vi "Main.vi"() -> ()   [LabVIEW 2020, in "SQSnobFit Control Panel.lvlib"]
uses:
  SQSnobFit Control Panel.lvlib
  process loops/Instrument Manager/Instrument State.ctl
  <vilib>/addons/zeromq/zmq_context.lvclass
  <vilib>/addons/zeromq/zmq_socket.lvclass
  process loops/UI Manager/support/Data Display Loop Data.ctl
  process loops/Logging/Logging Configuration.ctl
  process loops/UI Manager/support/UI Data.ctl
  process loops/UI Manager/support/UI Display State.ctl
  Typedefs/System Control Data.ctl
  <vilib>/Utility/error.llb/Error Cluster From Error Code.vi
  <vilib>/ErrorRing/Error Ring.xnode
  support/Message Queue/Message Queue.lvlib
  support/User Event - Stop/User Event - Stop.lvlib
  process loops/Instrument Manager/Instrument Manager.lvlib
  process loops/Acquisition/Acquisition.lvlib
  process loops/Remote Connection Manager/Remote Connection Manager.lvlib
  process loops/Logging/Logging.lvlib
panel:
  out "Next suggested parameters (percent)":cluster{"Name":string, "Value":dbl}[](array[cluster])
  in  "Overall Flow Rate (mL/min)":dbl format="%.3f"
  out "Next suggested parameters (values)":cluster{"Name":string, "Value":dbl}[](array[cluster])
  out "Response":string
  out "Optimizer Path":path
  in  "Time Interval (sec)":i32=1200
  out "Data Graph":cluster{timestamp[], dbl[]}[](graph)
  in  "Config Log Btn":bool
  in  "Sampling rate\n(sec/sample)":dbl=1.0 min=0.1 step=0.1
  in  "Log Data":bool
  in  "Submit Btn":bool
  in  "Yield":dbl format="%.3f"
  # "SQSnobFit"
  # "Optimizer Control"
  # "Config"
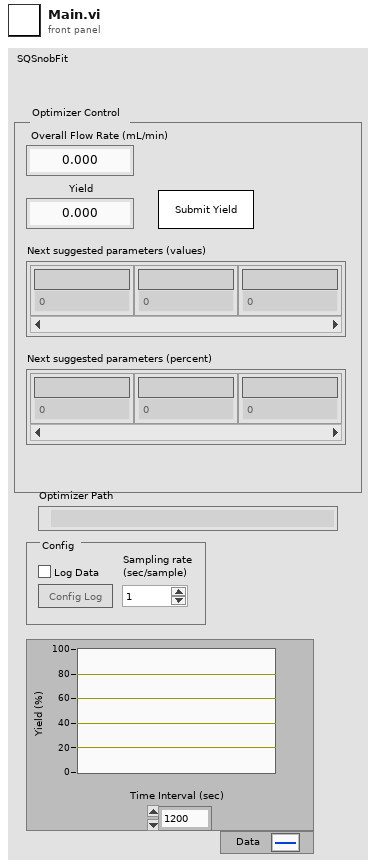
[diagram p1: front panel]
types:
  T1 = typedef "SQSnobFit Control Panel.lvlib/Data Display Loop Data.ctl" = cluster{"Data Timestamps":timestamp[], "Data Values":dbl[], "Previous Run State":bool}
  T2 = typedef "SQSnobFit Control Panel.lvlib/Instrument Manager.lvlib/Instrument State.ctl" = cluster{"Context":refnum<class "zmq_context.lvclass">, "Socket":refnum<class "zmq_socket.lvclass">, "Running Since":timestamp, "New Parameters (values)":cluster{"Time Stamp":timestamp, "Name":string[], "Value":dbl[]}, "Optimizer Path":path, "Running":bool, "Response Counter":u8, "Response Timeout (ms)":u32, "Response Retries":u32, "Endpoint":string, "Starting up?":bool, "New Parameters (percents)":cluster{"Time Stamp":timestamp, "Name":string[], "Value":dbl[]}, "Flow Rate Constant":dbl, "Yield":dbl, "Current Best (values)":cluster{"Parameter Names":string[], "Parameter Values":dbl[], "Function Value":dbl}}
  T3 = typedef "SQSnobFit Control Panel.lvlib/Message Queue.lvlib/All Message Queues.ctl" = cluster{"System Control":refnum<queue>, "Instrument":refnum<queue>, "Remote":refnum<queue>, "UI":refnum<queue>, "Acquisition":refnum<queue>, "Logging":refnum<queue>}
  T4 = typedef "SQSnobFit Control Panel.lvlib/UI Display State.ctl" = enum16{"Shown", "Hidden"}
  T5 = enum8{"Enabled", "Disabled", "Disabled and Grayed Out"}
  T6 = typedef "SQSnobFit Control Panel.lvlib/UI Data.ctl" = cluster{"Setpoint Ctl":refnum<vi>, "Submit Btn":refnum<vi>, "Log Data":refnum<vi>, "Config Log Btn":refnum<vi>, "Data Graph":refnum<vi>, "Flow Rate Ctl":refnum<vi>}
  T7 = typedef "SQSnobFit Control Panel.lvlib/Logging.lvlib/Logging Configuration.ctl" = cluster{"Log Directory Path":path, "Log File Path":path, "Log File Prefix":string, "Log File Extension":string, "File Delimiter":string, "Header Info":string[][], "Channels":string[], "Log Instrument Runs":bool}
  T8 = typedef "SQSnobFit Control Panel.lvlib/System Control Data.ctl" = cluster{"Example Value <Replace Me>":dbl, "Log Runs":bool, "Clone":bool}
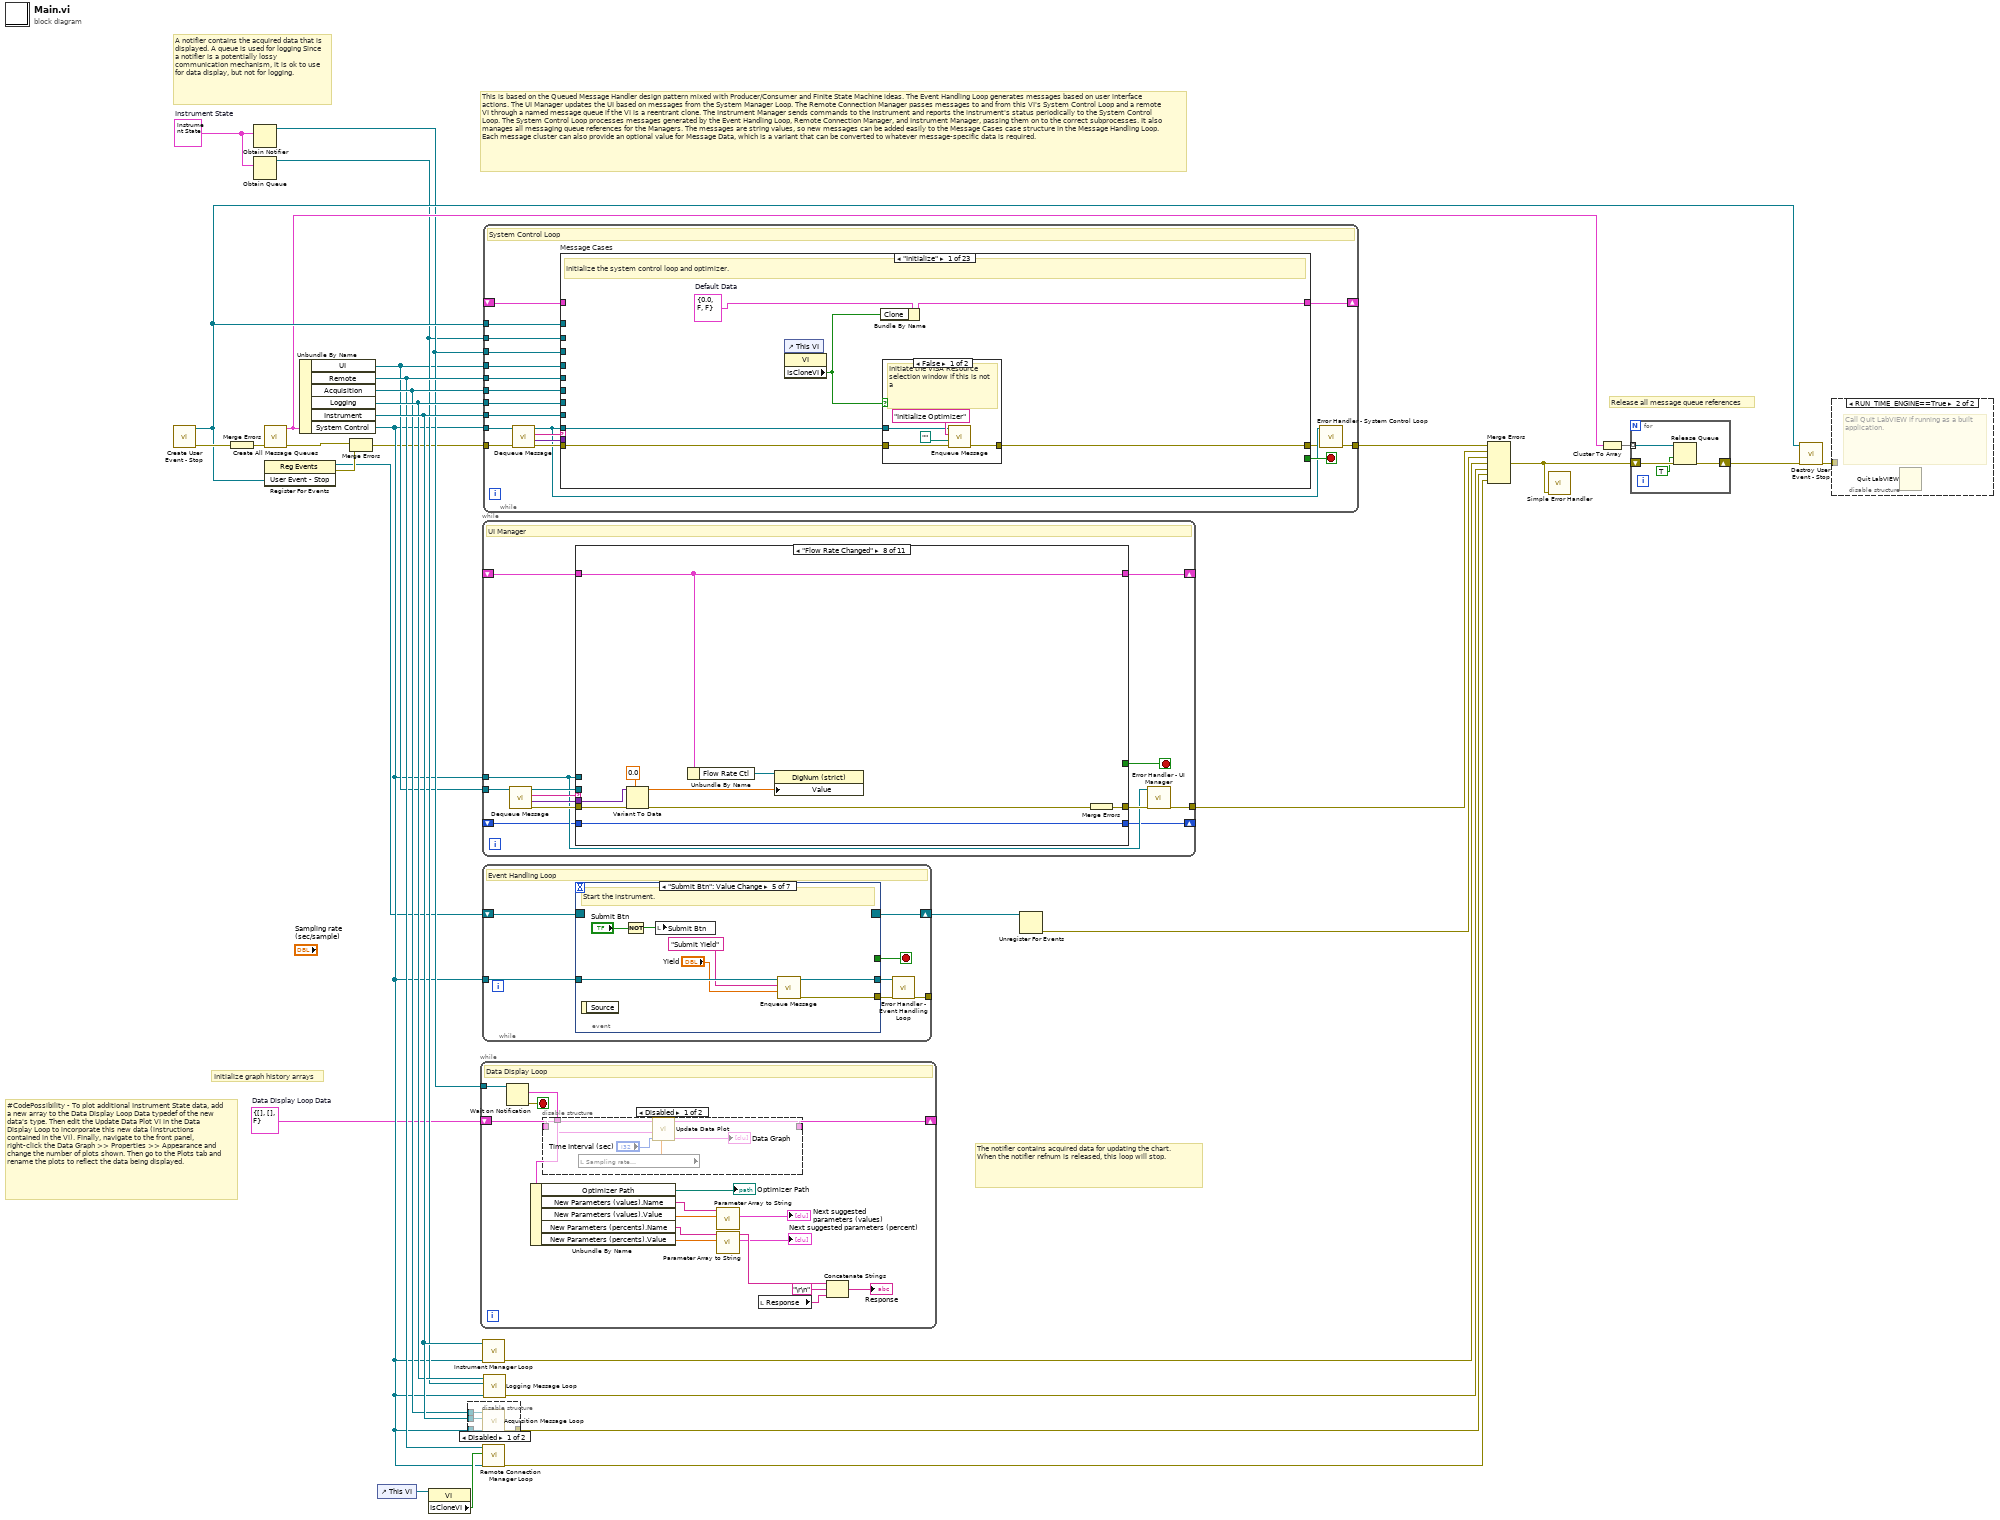
[diagram p0: block diagram]
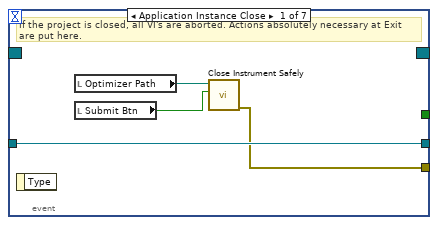
[diagram p4: hidden frame]
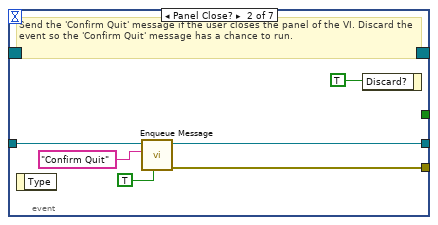
[diagram p5: hidden frame]
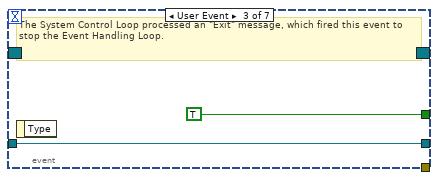
[diagram p6: hidden frame]
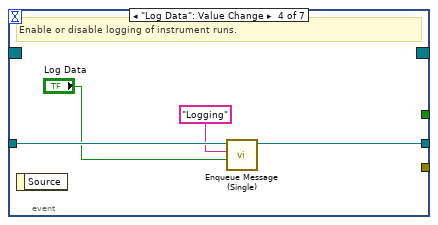
[diagram p7: hidden frame]
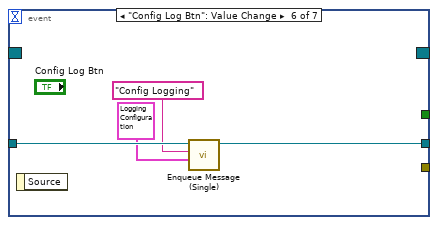
[diagram p8: hidden frame]
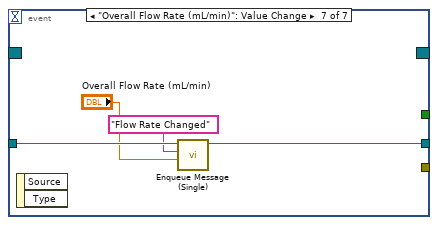
[diagram p9: hidden frame]
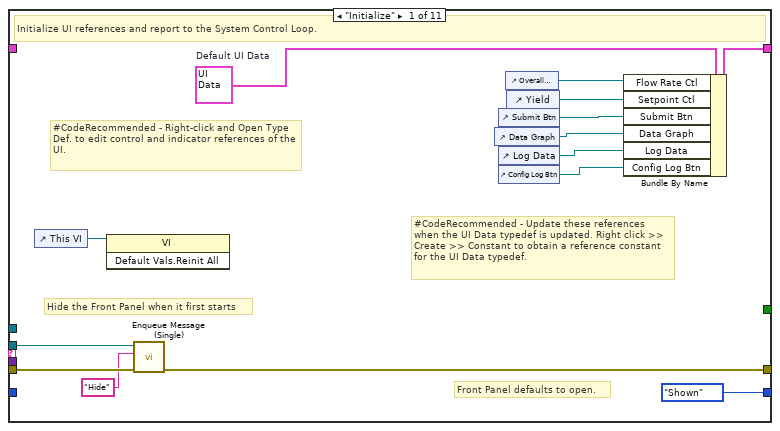
[diagram p10: hidden frame]
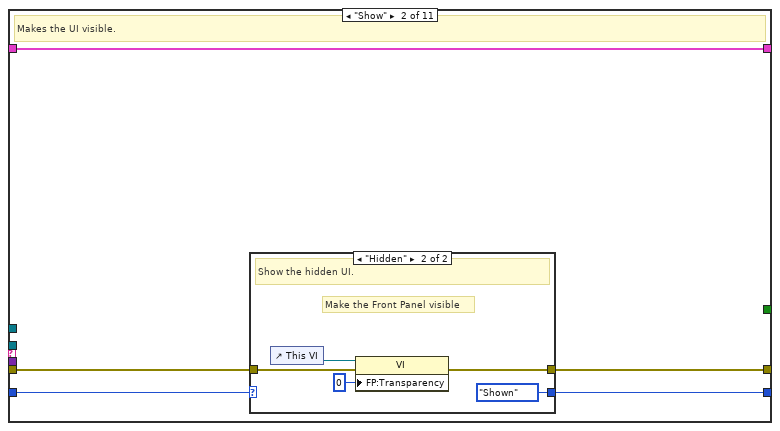
[diagram p11: hidden frame]
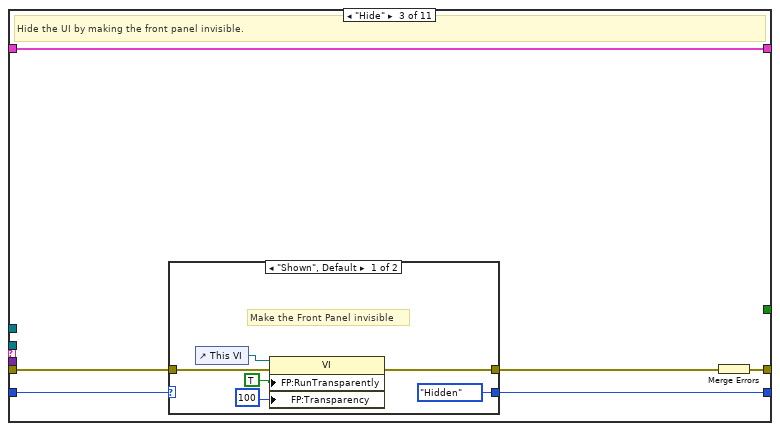
[diagram p13: hidden frame]
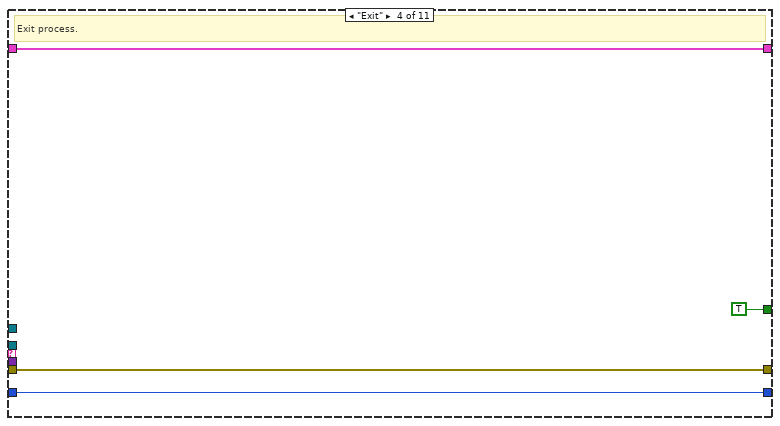
[diagram p15: hidden frame]
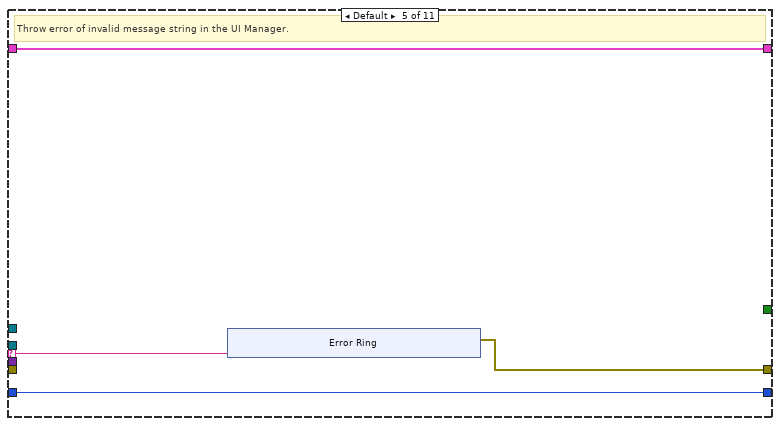
[diagram p16: hidden frame]
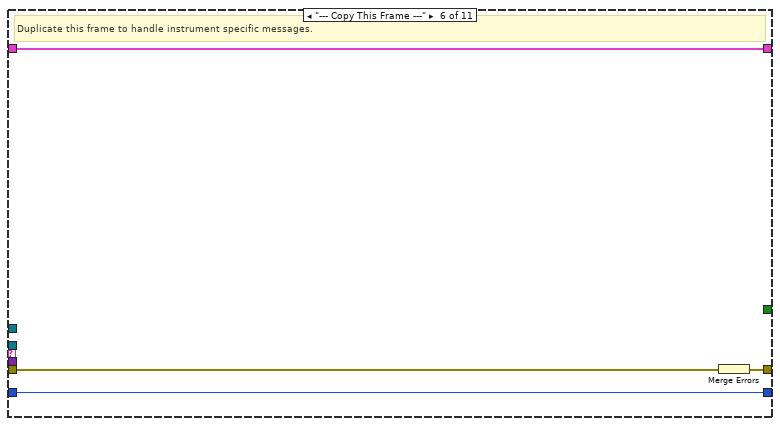
[diagram p17: hidden frame]
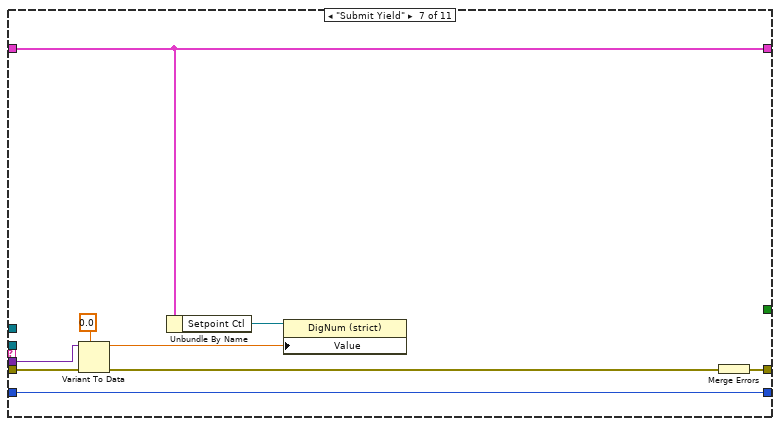
[diagram p18: hidden frame]
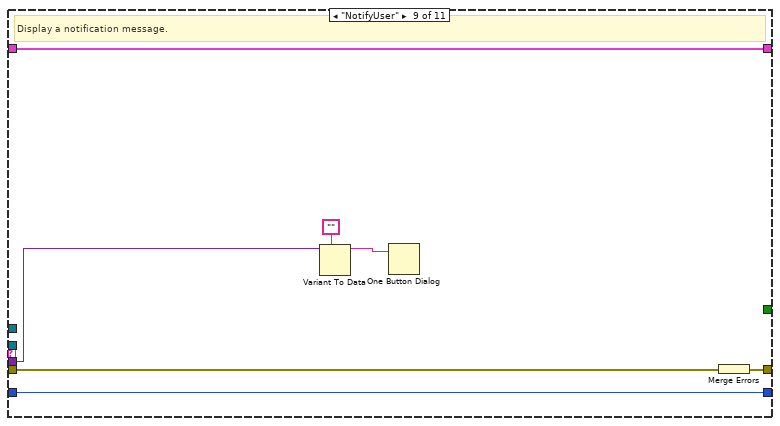
[diagram p19: hidden frame]
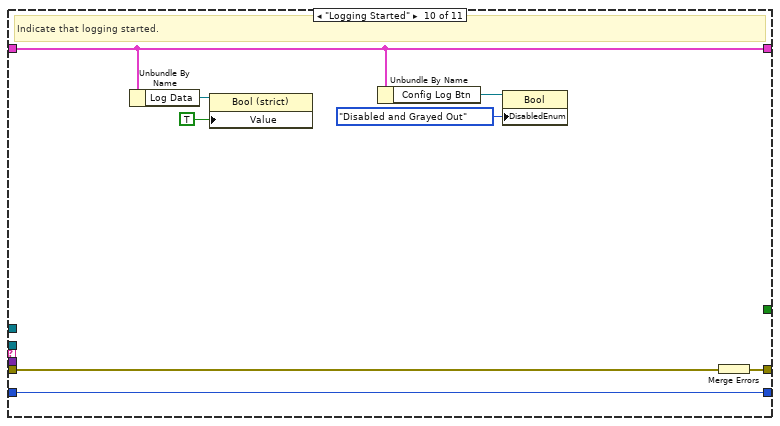
[diagram p20: hidden frame]
diagram:
  w2 = T1 {"Data Timestamps"=[], "Data Values"=[], "Previous Run State"=FALSE}  # Data Display Loop Data
  w1 = T2 {"Context"=refnum, "Socket"=refnum, "Running Since"=timestamp(0 s since 1904-01-01), "New Parameters (values)"={"Time Stamp"=timestamp(0 s since 1904-01-01), "Name"=[], "Value"=[]}, "Optimizer Path"=path "", "Running"=FALSE, "Response Counter"=0, "Response Timeout (ms)"=0, "Response Retries"=0, "Endpoint"="", "Starting up?"=FALSE, "New Parameters (percents)"={"Time Stamp"=timestamp(0 s since 1904-01-01), "Name"=[], "Value"=[]}, "Flow Rate Constant"=0.0, "Yield"=0.0, "Current Best (values)"={"Parameter Names"=[], "Parameter Values"=[], "Function Value"=0.0}}  # Instrument State
  # "#CodePossibility - To plot additional Instrument State data, add a new array to the Data Display Loop Data typedef of the new data's type. Then edit the Update Data Plot VI in the Data Display Loop to incorporate this new data (instructions contained in the VI). Finally, navigate to the front panel, right-click the Data Graph >> Properties >> Appearance and change the number of plots shown. Then go to the Plots tab and rename the plots to reflect the data being displayed."
  # "Initialize graph history arrays"
  # "A notifier contains the acquired data that is displayed. A queue is used for logging Since a notifier is a potentially lossy communication mechanism, it is ok to use for data display, but not for logging."
  # "The notifier contains acquired data for updating the chart. When the notifier refnum is released, this loop will stop."
  # "Release all message queue references"
  # "This is based on the Queued Message Handler design pattern mixed with Producer/Consumer and Finite State Machine ideas. The Event Handling Loop generates messages based on user interface actions. The UI Manager updates the UI based on messages from the System Manager Loop. The Remote Connection Manager passes messages to and from this VI's System Control Loop and a remote VI through a named message queue if the VI is a reentrant clone. The Instrument Manager sends commands to the instrument and reports the instrument's status periodically to the System Control Loop. The System Control Loop processes messages generated by the Event Handling Loop, Remote Connection Manager, and Instrument Manager, passing them on to the correct subprocesses. It also manages all messaging queue references for the Managers. The messages are string values, so new messages can be added easily to the Message Cases case structure in the Message Handling Loop.  Each message cluster can also provide an optional value for Message Data, which is a variant that can be converted to whatever message-specific data is required."
  n1 = call "Create User Event - Stop.vi"() -> ("error out"=w26:errorcluster, "User Event - Stop"=w22:refnum<user-event>)  [unwired: 10 in]
  n2 = Merge Errors(w26) -> (w25:errorcluster)
  n3 = Obtain Notifier(notification data type=w1) -> (notifier out=w8:refnum<notifier>)  [unwired: 3 in, 2 out]
  n4 = Obtain Queue(element data type=w1) -> (queue out=w7:refnum<queue>)  [unwired: 4 in, 2 out]
  n5 = call "Create All Message Queues.vi"("error in (no error)"=w25) -> ("error out"=w28:errorcluster, "Message Queues out"=w11:T3)  [unwired: 9 in]
  n6 = register-events(w22) -> (reference out=w3:refnum<event-registration>, error out=w13:errorcluster)  [unwired: 2 in]
  n7 = Unbundle By Name(w11) -> ("UI"=w6:refnum<queue>, "Remote"=w29:refnum<queue>, "Acquisition"=w30:refnum<queue>, "Logging"=w31:refnum<queue>, "Instrument"=w32:refnum<queue>, "System Control"=w5:refnum<queue>)
  n8 = Merge Errors(w28, w13) -> (w4:errorcluster)
  n9 = control-ref of="This VI"() -> (w21:refnum<vi>)
  n10 = property class="VI"(reference=w21) -> ("IsCloneVI"=w20:bool)  [unwired: 1 in, 2 out]
  n11 = disable-structure shown="Disabled" {
    disable-tunnel: w32 -> [w36 _]
    disable-tunnel: w30 -> [w35 _]
    disable-tunnel: [w34 _] -> w15
    disable-tunnel: w5 -> [w33 _]
    frame Disabled {
      n12 = call "Acquisition Message Loop.vi"("System Control"=w33, "Instrument Manager"=w36, "Acquisition"=w35) -> ("error out"=w34:errorcluster)  [unwired: 8 in]
    }
    frame Enabled {
    }
  }
  n13 = while "Data Display Loop" {
    tunnel: w8 -> [w52]
    shift-right: [w49] -> _
    shift-left: w2 -> [w50]
    stop <- w51 stop-if-true
    # "Data Display Loop"
    n14 = Wait on Notification(notifier=w52) -> (notification=w48:T2, error out=w51:errorcluster)  [unwired: 3 in, 2 out]
    n15 = Unbundle By Name(w48) -> ("Optimizer Path"=→"Optimizer Path":path, "New Parameters (values).Name"=w43:string[], "New Parameters (values).Value"=w42:dbl[], "New Parameters (percents).Name"=w40:string[], "New Parameters (percents).Value"=w39:dbl[])
    n16 = disable-structure shown="Disabled" {
      disable-tunnel: w50 -> [w58 _]
      disable-tunnel: [w57 _] -> w49
      disable-tunnel: w48 -> [w56 _]
      frame Disabled {
        n17 = local read "Sampling rate\n(sec/sample)"() -> (w53:dbl)
        n18 = call "Update Data Plot.vi"("Sample Rate (sec/sample)"=w53, "Time interval (s)"="Time Interval (sec)", "Optimizer State"=w56, "Graph History Arrays in"=w58) -> ("Updated Graph History"=→"Data Graph":cluster{timestamp[], dbl[]}[], "Graph History Arrays out"=w57:T1)  [unwired: 6 in]
      }
      frame Enabled {
      }
    }
    n19 = call "Parameter Array to String.vi"("Parameter Values"=w42, "Parameter Labels"=w43) -> ("Parameter Array"=→"Next suggested parameters (values)":cluster{"String":string, "Numeric":dbl}[])  [unwired: 8 in, 1 out]
    n20 = call "Parameter Array to String.vi"("Parameter Values"=w39, "Parameter Labels"=w40) -> ("Parameter Array"=→"Next suggested parameters (percent)":cluster{"String":string, "Numeric":dbl}[], "Parameter String"=w38:string)  [unwired: 8 in]
    n21 = local read "Response"() -> (w44:string)
    n22 = Concatenate Strings(w38, "\r\n", w44) -> (→"Response":string)
  }
  n23 = while {
    tunnel: w6 -> [w71]
    tunnel: w5 -> [w62]
    tunnel: [w63] -> w19
    shift-right: [w66] -> _
    shift-left: _ -> [w65]
    shift-right: [w60] -> _
    shift-left: _ -> [w59]
    stop <- w61 stop-if-true
    # "UI Manager"
    n24 = call "Dequeue Message.vi"("Message Queue"=w71) -> ("error out"=w69:errorcluster, "Message Data"=w67:variant, "Message"=w68:string, "dup Message Queue"=w70:refnum<queue>)  [unwired: 7 in]
    n25 = case shown="\"Flow Rate Changed\"" w68 {
      selector: w68 -> [_ _ _ _ w119 _ _ _ _ _ _]
      tunnel: w70 -> [w79 _ _ _ _ _ _ _ _ _ _]
      tunnel: w69 -> [w82 w89 w101 w115 _ w128 w138 w147 w153 w162 w170]
      tunnel: w67 -> [_ _ _ _ _ _ w133 w142 w151 _ _]
      tunnel: w62 -> [_ _ _ _ _ _ _ _ _ _ _]
      tunnel: [w80 w88 w102 w115 w118 w129 w139 w148 w154 w163 w171] -> w64
      tunnel: [w84 w90 w103 w114 w117 w130 w136 w145 w155 w158 w164] -> w66
      tunnel: w65 -> [_ w90 w103 w114 w117 w130 w136 w145 w155 w158 w164]
      tunnel: [_ _ _ TRUE _ _ _ _ _ _ _] -> w61
      tunnel: w59 -> [_ w87 w99 w112 w116 w127 w137 w146 w152 w161 w169]
      tunnel: [UI_Display_State."Shown" ("UI Display State") w86 w98 w112 w116 w127 w137 w146 w152 w161 w169] -> w60
      frame "Initialize" {
        w85 = T6 {"Setpoint Ctl"=refnum, "Submit Btn"=refnum, "Log Data"=refnum, "Config Log Btn"=refnum, "Data Graph"=refnum, "Flow Rate Ctl"=refnum}  # Default UI Data
        # "Front Panel defaults to open."
        # "Hide the Front Panel when it first starts"
        # "#CodeRecommended - Update these references when the UI Data typedef is updated. Right click >> Create >> Constant to obtain a reference constant for the UI Data typedef."
        # "#CodeRecommended - Right-click and Open Type Def. to edit control and indicator references of the UI."
        # "Initialize UI references and report to the System Control Loop."
        n26 = control-ref of="This VI"() -> (w76:refnum<vi>)
        n27 = invoke class="VI" method="Default Vals.Reinit All"(reference=w76) -> ()  [unwired: 2 in, 3 out]
        n28 = call "Enqueue Message (Single).vi"("error in (no error)"=w82, "Message"="Hide", "Message Queue"=w79) -> ("error out"=w80:errorcluster)  [unwired: 7 in, 1 out]
        n29 = control-ref of="Data Graph"() -> (w75:refnum<vi>)
        n30 = control-ref of="Submit Btn"() -> (w81:refnum<vi>)
        n31 = control-ref of="Log Data"() -> (w74:refnum<vi>)
        n32 = control-ref of="Config Log Btn"() -> (w73:refnum<vi>)
        n33 = control-ref of="Overall Flow Rate (mL/min)"() -> (w72:refnum<vi>)
        n34 = control-ref of="Yield"() -> (w83:refnum<vi>)
        n35 = Bundle By Name(cluster=w85, "Flow Rate Ctl"=w72, "Setpoint Ctl"=w83, "Submit Btn"=w81, "Data Graph"=w75, "Log Data"=w74, "Config Log Btn"=w73) -> (w84:T6)
      }
      frame "Show" {
        # "Makes the UI visible."
        n36 = case shown="\"Hidden\"" w87 {
          selector: w87 -> [w92 _]
          tunnel: w89 -> [w91 w97]
          tunnel: [w91 w95] -> w88
          tunnel: [w92 UI_Display_State."Shown" ("UI Display State")] -> w86
          frame "Shown", Default {
            # "Do nothing if UI is already shown."
          }
          frame "Hidden" {
            # "Make the Front Panel visible"
            # "Show the hidden UI."
            n37 = control-ref of="This VI"() -> (w96:refnum<vi>)
            n38 = property class="VI"(reference=w96, error in=w97, "FP:Transparency"=u8 0 ("Front Panel Window:Transparency")) -> (error out=w95:errorcluster)  [unwired: 1 out]
          }
        }
      }
      frame "Hide" {
        # "Hide the UI by making the front panel invisible."
        n39 = case shown="\"Shown\", Default" w99 {
          selector: w99 -> [_ w111]
          tunnel: w101 -> [w106 w110]
          tunnel: [w105 w110] -> w100
          tunnel: [UI_Display_State."Hidden" ("UI Display State") w111] -> w98
          frame "Shown", Default {
            # "Make the Front Panel invisible"
            n40 = control-ref of="This VI"() -> (w109:refnum<vi>)
            n41 = property class="VI"(reference=w109, error in=w106, "FP:RunTransparently"=TRUE ("Front Panel Window:Run VI Transparently"), "FP:Transparency"=u8 100 ("Front Panel Window:Transparency")) -> (error out=w105:errorcluster)  [unwired: 1 out]
          }
          frame "Hidden" {
          }
        }
        n42 = Merge Errors(w100) -> (w102:errorcluster)
      }
      frame "Exit" {
        # "Exit process."
      }
      frame Default {
        # "Throw error of invalid message string in the UI Manager."
        n43 = xnode "Error Ring"("parameter 0"=w119) -> ("error out"=w118:errorcluster)
      }
      frame "--- Copy This Frame ---" {
        # "Duplicate this frame to handle instrument specific messages."
        n44 = Merge Errors(w128) -> (w129:errorcluster)
      }
      frame "Submit Yield" {
        n45 = Variant To Data(error in=w138, type=0.0, Variant=w133) -> (data=w131:dbl, error out=w134:errorcluster)
        n46 = Unbundle By Name(w136) -> ("Setpoint Ctl"=w135:refnum<vi>)
        n47 = property class="DigNum (strict)"(reference=w135, "Value"=w131) -> ()  [unwired: 1 in, 2 out]
        n48 = Merge Errors(w134) -> (w139:errorcluster)
      }
      frame "Flow Rate Changed" {
        n49 = Variant To Data(error in=w147, type=0.0, Variant=w142) -> (data=w140:dbl, error out=w143:errorcluster)
        n50 = Unbundle By Name(w145) -> ("Flow Rate Ctl"=w144:refnum<vi>)
        n51 = property class="DigNum (strict)"(reference=w144, "Value"=w140) -> ()  [unwired: 1 in, 2 out]
        n52 = Merge Errors(w143) -> (w148:errorcluster)
      }
      frame "NotifyUser" {
        # "Display a notification message."
        n53 = Variant To Data(type="", Variant=w151) -> (data=w149:string)  [unwired: 1 in, 1 out]
        n54 = One Button Dialog(message=w149) -> ()  [unwired: 1 in, 1 out]
        n55 = Merge Errors(w153) -> (w154:errorcluster)
      }
      frame "Logging Started" {
        # "Indicate that logging started."
        n56 = Unbundle By Name(w158) -> ("Log Data"=w160:refnum<vi>)
        n57 = property class="Bool (strict)"(reference=w160, "Value"=TRUE ("Log Data")) -> ()  [unwired: 1 in, 2 out]
        n58 = Unbundle By Name(w158) -> ("Config Log Btn"=w157:refnum<vi>)
        n59 = property class="Bool"(reference=w157, "DisabledEnum"=T5."Disabled and Grayed Out" ("Disabled")) -> ()  [unwired: 1 in, 2 out]
        n60 = Merge Errors(w162) -> (w163:errorcluster)
      }
      frame "Logging Stopped" {
        # "Indicate that logging stopped."
        n61 = Unbundle By Name(w164) -> ("Log Data"=w168:refnum<vi>)
        n62 = property class="Bool (strict)"(reference=w168, "Value"=FALSE ("Log Data")) -> ()  [unwired: 1 in, 2 out]
        n63 = Unbundle By Name(w164) -> ("Config Log Btn"=w166:refnum<vi>)
        n64 = property class="Bool"(reference=w166, "DisabledEnum"=T5."Enabled" ("Disabled")) -> ()  [unwired: 1 in, 2 out]
        n65 = Merge Errors(w170) -> (w171:errorcluster)
      }
    }
    n66 = call "Error Handler - UI Manager.vi"("error in (no error)"=w64, "Message Queue"=w62) -> ("dup error in"=w63:errorcluster)  [unwired: 8 in, 1 out]
  }
  n67 = while {
    tunnel: w5 -> [w178]
    shift-right: [w176] -> w23
    shift-left: w3 -> [w177]
    tunnel: [w172] -> _
    stop <- w174 stop-if-true
    # "Event Handling Loop"
    n68 = event shown="[4] \"Submit Btn\": Value Change" {
      selector: w177 -> [_ _ _ _ _ _ _]
      dyn-events: [_ _ _ _ _ _ _] -> w176
      timeout: _ -> [_ _ _ _ _ _ _]
      tunnel: [_ _ TRUE ("Discard?") _ _ _ _] -> w174
      tunnel: w178 -> [w182 w187 w190 w194 w201 w205 w209]
      tunnel: [w181 w186 _ _ w199 _ _] -> w175
      tunnel: [w182 w185 w190 w193 w200 w204 w208] -> w173
      event Application Instance Close {
        # "If the project is closed, all VI's are aborted. Actions absolutely necessary at Exit are put here."
        n69 = event-data() -> ()  [unwired: 1 in, 1 out]
        n70 = local read "Optimizer Path"() -> (w179:path)
        n71 = local read "Submit Btn"() -> (w180:bool)
        n72 = call "Close Instrument Safely.vi"("Running (F)"=w180, "Optimizer Path"=w179) -> ("error out"=w181:errorcluster)  [unwired: 9 in]
      }
      event Panel Close? {
        # "Send the 'Confirm Quit' message if the user closes the panel of the VI. Discard the event so the 'Confirm Quit' message has a chance to run."
        n73 = event-data() -> ()  [unwired: 1 in, 1 out]
        n74 = call-poly "Enqueue Message.vi"("Priority Message? (F)"=TRUE, "Message"="Confirm Quit", "Message Queue"=w187) -> ("error out"=w186:errorcluster, "dup Message Queue"=w185:refnum<queue>)  [unwired: 7 in]
        n75 = event-data("Discard?"=TRUE) -> ()  [unwired: 1 in, 1 out]
      }
      event User Event {
        # "The System Control Loop processed an \"Exit\" message, which fired this event to stop the Event Handling Loop."
        n76 = event-data() -> ()  [unwired: 1 in, 1 out]
      }
      event "Log Data": Value Change {
        # "Enable or disable logging of instrument runs."
        n77 = event-data() -> ()  [unwired: 1 in, 1 out]
        n78 = call "Enqueue Message (Single).vi"("Message Data"="Log Data", "Message"="Logging", "Message Queue"=w194) -> ("dup Message Queue"=w193:refnum<queue>)  [unwired: 7 in, 1 out]
      }
      event "Submit Btn": Value Change {
        # "Start the instrument."
        n79 = event-data() -> ()  [unwired: 1 in, 1 out]
        n80 = Not(x="Submit Btn") -> (.not. x?=w195:bool)
        n81 = local write "Submit Btn"(w195) -> ()
        n82 = call-poly "Enqueue Message.vi"("Message Data"="Yield", "Message"="Submit Yield", "Message Queue"=w201) -> ("error out"=w199:errorcluster, "dup Message Queue"=w200:refnum<queue>)  [unwired: 7 in]
      }
      event "Config Log Btn": Value Change {
        n83 = event-data() -> ()  [unwired: 1 in, 1 out]
        n84 = call "Enqueue Message (Single).vi"("Message Data"=T7 {"Log Directory Path"=path "", "Log File Path"=path "", "Log File Prefix"="Experiment", "Log File Extension"="csv", "File Delimiter"=",", "Header Info"=[], "Channels"=[], "Log Instrument Runs"=FALSE} ("Logging Configuration"), "Message"="Config Logging", "Message Queue"=w205) -> ("dup Message Queue"=w204:refnum<queue>)  [unwired: 7 in, 1 out]
      }
      event "Overall Flow Rate (mL/min)": Value Change {
        n85 = event-data() -> ()  [unwired: 1 in, 2 out]
        n86 = call "Enqueue Message (Single).vi"("Message Data"="Overall Flow Rate (mL/min)", "Message"="Flow Rate Changed", "Message Queue"=w209) -> ("dup Message Queue"=w208:refnum<queue>)  [unwired: 7 in, 1 out]
      }
    }
    n87 = call "Error Handler - Event Handling Loop.vi"("error in (no error)"=w175, "Message Queue"=w173) -> ("dup error in"=w172:errorcluster)  [unwired: 8 in, 1 out]
  }
  n88 = call "Instrument Manager Loop.vi"("System Control"=w5, "Optimizer Manager"=w32) -> ("error out"=w17:errorcluster)  [unwired: 9 in]
  n89 = call "Remote Connection Manager Loop.vi"("System Control"=w5, "IsCloneVI (false)"=w20, "Remote"=w29) -> ("error out"=w14:errorcluster)  [unwired: 8 in]
  n90 = while {
    tunnel: w5 -> [w220]
    shift-right: [w227] -> _
    shift-left: _ -> [w228]
    tunnel: w22 -> [w225]
    tunnel: w4 -> [w224]
    tunnel: [w218] -> w27
    tunnel: w32 -> [w216]
    tunnel: w29 -> [w215]
    tunnel: w6 -> [w214]
    tunnel: w30 -> [w213]
    tunnel: w31 -> [w212]
    tunnel: w8 -> [w211]
    tunnel: w7 -> [w210]
    stop <- w226 stop-if-true
    # "System Control Loop"
    n91 = call "Dequeue Message.vi"("error in (no error)"=w224, "Message Queue"=w220) -> ("error out"=w223:errorcluster, "Message Data"=w221:variant, "Message"=w222:string, "dup Message Queue"=w219:refnum<queue>)  [unwired: 6 in]
    n92 = case "Message Cases" shown="\"Initialize\"" w222 {
      selector: w222 -> [_ _ _ w270 w283 w294 w312 w327 w341 w347 w378 _ _ w418 w425 w432 w439 w446 w456 w470 w486 w500 w513]
      tunnel: w219 -> [w231 _ w250 _ _ _ _ _ _ _ _ w389 _ _ _ _ _ _ _ _ _ _ _]
      tunnel: w223 -> [w230 w247 w254 _ _ w297 w315 w330 w345 w363 w382 w393 w401 w422 w429 w436 w443 w450 w459 w473 w490 w504 _]
      tunnel: [w229 w241 w252 w273 w284 w303 w317 w332 w346 w354 w380 w391 w406 w423 w430 w437 w444 w451 w460 w474 w488 w502 w524] -> w217
      tunnel: w228 -> [_ w246 w253 w269 w285 w304 w318 w333 w344 w353 w381 w392 w407 w424 w431 w438 w445 w452 w461 w475 w489 w503 w522]
      tunnel: [w233 w246 w253 w269 w285 w304 w318 w333 w344 w353 w381 w392 w405 w424 w431 w438 w445 w452 w461 w475 w489 w503 w522] -> w227
      tunnel: [_ _ _ TRUE _ _ _ _ _ _ _ _ _ _ _ _ _ _ _ _ _ _ _] -> w226
      tunnel: w221 -> [_ w245 _ w274 _ w293 w311 w326 w340 w348 w379 _ w403 w419 w426 w433 w440 w447 w457 w471 w485 w499 w514]
      tunnel: w225 -> [_ _ _ w271 _ _ _ _ _ _ _ _ _ _ _ _ _ _ _ _ _ _ _]
      tunnel: w216 -> [_ _ _ w266 _ w298 _ _ w342 _ _ _ _ _ _ _ _ _ _ _ w481 w496 _]
      tunnel: w215 -> [_ _ _ w265 _ w301 w316 w325 _ w358 w375 _ _ _ _ _ _ _ w455 w469 _ _ w523]
      tunnel: w214 -> [_ _ _ w264 _ w300 _ w331 _ w357 _ _ _ _ _ _ _ _ w454 w468 w482 w497 _]
      tunnel: w213 -> [_ _ _ w268 _ w302 _ _ _ w360 w377 _ _ _ _ _ _ _ _ _ w484 _ _]
      tunnel: w212 -> [_ _ _ w267 _ w299 _ _ _ w350 w376 _ w399 w420 w427 w434 w441 w448 _ _ _ _ w512]
      tunnel: w211 -> [_ _ _ w261 _ _ _ _ _ _ _ _ _ _ _ _ _ _ _ _ _ _ w521]
      tunnel: w210 -> [_ _ _ w259 _ _ _ _ _ _ _ _ _ _ _ _ _ _ _ _ _ _ w518]
      frame "Initialize" {
        w234 = T8 {"Example Value <Replace Me>"=0.0, "Log Runs"=FALSE, "Clone"=FALSE}  # Default Data
        # "Initialize the system control loop and optimizer."
        n93 = control-ref of="This VI"() -> ()  [unwired: 1 out]
        n94 = property on="Property Node" class="VI"() -> ("IsCloneVI"=w232:bool)  [unwired: 2 in, 2 out]
        n95 = Bundle By Name(cluster=w234, "Clone"=w232) -> (w233:T8)
        n96 = case shown="False" w232 {
          tunnel: w230 -> [w237 w240]
          tunnel: [w236 w240] -> w229
          tunnel: w231 -> [w235 _]
          frame False {
            # "Initiate the VISA Resource selection window if this is not a"
            n97 = call-poly "Enqueue Message.vi"("error in (no error)"=w237, "Message Data"=path "" ("VISA resource out"), "Message"="Initialize Optimizer", "Message Queue"=w235) -> ("error out"=w236:errorcluster)  [unwired: 6 in, 1 out]
          }
          frame True {
            # "Reentrant clone. It is the responsibility of the RCM to send the Set VISA Resource command."
          }
        }
      }
      frame "Error" {
        # "#CodeRecommended - If you ever change the name of this \"Error\" message, you'll need to update the name in the Check Loop Error.vi as well."
        # "#CodeRecommended - Consider creating a system for logging errors in some way. These errors are for notification purposes only. Handling of specific errors should be performed in the message frames that generated the error."
        # "Error - Display an error dialog. This message is sent by the \"Error Handler\" VIs at the end of other loops in this application."
        n98 = Variant To Data(error in=w247, type=errorcluster {"status"=FALSE, "code"=0, "source"=""} ("error constant"), Variant=w245) -> (data=w243:errorcluster, error out=w242:errorcluster)
        n99 = call <vilib>:"Simple Error Handler.vi"("error in (no error)"=w243) -> ()  [unwired: 4 in, 5 out]
        n100 = Merge Errors(w242) -> (w241:errorcluster)
      }
      frame "Confirm Quit" {
        # "#CodeNeeded - If you want to provide an \"Are you sure\" dialog (or some other notification) before the application exits, place that code here. This message is typically sent from a Panel Close? event."
        # "Confirm Quit - Message that can confirm whether or not the user wants to exit the application."
        n101 = call-poly "Enqueue Message.vi"("Priority Message? (F)"=TRUE, "error in (no error)"=w254, "Message"="Exit", "Message Queue"=w250) -> ("error out"=w251:errorcluster)  [unwired: 6 in, 1 out]
        n102 = Merge Errors(w251) -> (w252:errorcluster)
      }
      frame "Exit" {
        # "Order other processes to exit"
        # "Begin the application closing procedure by sending \"Exit\" commands to all running processes."
        n103 = Variant To Data(type=errorcluster {"status"=FALSE, "code"=0, "source"=""} ("error constant"), Variant=w274) -> (data=w275:errorcluster)  [unwired: 1 in, 1 out]
        n104 = Build Array(w264, w265, w268, w267, w266) -> (w263:refnum<queue>[])
        n105 = call <vilib>:"Clear Errors.vi"("error in (no error)"=w275, "specific error code to clear (0: all)"=5000) -> ("error out"=w256:errorcluster)  [unwired: 4 in, 1 out]
        n106 = call <vilib>:"Simple Error Handler.vi"("error in (no error)"=w256) -> ()  [unwired: 4 in, 5 out]
        n107 = for {
          tunnel: w270 -> [w281]
          tunnel: w263 -> [w280] mode=indexing
          shift-right: [w279] -> w272
          shift-left: _ -> [w278]
          n108 = call "Enqueue Message (Single).vi"("Priority Message? (F)"=TRUE, "Message"=w281, "Message Queue"=w280) -> ("error out"=w282:errorcluster)  [unwired: 7 in, 1 out]
          n109 = Merge Errors(w282, w278) -> (w279:errorcluster)
        }
        n110 = Release Notifier(notifier=w261) -> (error out=w260:errorcluster)  [unwired: 2 in, 2 out]
        n111 = Release Queue(queue=w259) -> (error out=w257:errorcluster)  [unwired: 2 in, 2 out]
        n112 = call "Fire User Event - Stop.vi"("User Event - Stop"=w271) -> ("error out"=w258:errorcluster)  [unwired: 10 in]
        n113 = Merge Errors(w258, w257, w260, w272) -> (w273:errorcluster)
      }
      frame Default {
        # "'Default' case only runs if there is a message that isn't defined in any of the other cases.  Output a programming error."
        n114 = xnode "Error Ring"("parameter 0"=w283) -> ("error out"=w284:errorcluster)
      }
      frame "---Copy This Frame---" {
        # "Sends the message to each process in the array."
        # "#CodeRecommended - Change connections to build an array of the processes that will receive this message"
        # "Duplicate this frame when creating new messages.  Change this comment in the duplicated frame to describe this message."
        n115 = Build Array(w300, w301, w302, w299, w298) -> (w295:refnum<queue>[])
        n116 = for {
          tunnel: w295 -> [w308] mode=indexing
          tunnel: w294 -> [w310]
          tunnel: w293 -> [w309]
          shift-right: [w307] -> w296
          shift-left: w297 -> [w305]
          n117 = call "Enqueue Message (Single).vi"("Message Data"=w309, "Message"=w310, "Message Queue"=w308) -> ("error out"=w306:errorcluster)  [unwired: 7 in, 1 out]
          n118 = Merge Errors(w306, w305) -> (w307:errorcluster)
        }
        n119 = Merge Errors(w296) -> (w303:errorcluster)
      }
      frame "Set Remote Queue" {
        # "Sends the message to each process in the array."
        # "Bounce this message back to the Remote Control Manager to set the remote queue to publish messages to."
        n120 = Build Array(w316) -> (w313:refnum<queue>[])
        n121 = for {
          tunnel: w313 -> [w322] mode=indexing
          tunnel: w312 -> [w324]
          tunnel: w311 -> [w323]
          shift-right: [w321] -> w314
          shift-left: w315 -> [w319]
          n122 = call "Enqueue Message (Single).vi"("Message Data"=w323, "Message"=w324, "Message Queue"=w322) -> ("error out"=w320:errorcluster)  [unwired: 7 in, 1 out]
          n123 = Merge Errors(w320, w319) -> (w321:errorcluster)
        }
        n124 = Merge Errors(w314) -> (w317:errorcluster)
      }
      frame "NotifyUser" {
        # "Sends the message to each process in the array."
        # "Forward notification messages to the UI Manager."
        n125 = Build Array(w331, w325) -> (w328:refnum<queue>[])
        n126 = for {
          tunnel: w328 -> [w337] mode=indexing
          tunnel: w327 -> [w339]
          tunnel: w326 -> [w338]
          shift-right: [w336] -> w329
          shift-left: w330 -> [w334]
          n127 = call "Enqueue Message (Single).vi"("Message Data"=w338, "Message"=w339, "Message Queue"=w337) -> ("error out"=w335:errorcluster)  [unwired: 7 in, 1 out]
          n128 = Merge Errors(w335, w334) -> (w336:errorcluster)
        }
        n129 = Merge Errors(w329) -> (w332:errorcluster)
      }
      frame "Initialize Optimizer" {
        # "Update the Optimizer path."
        n130 = call "Enqueue Message (Single).vi"("error in (no error)"=w345, "Message Data"=w340, "Message"=w341, "Message Queue"=w342) -> ("error out"=w343:errorcluster)  [unwired: 6 in, 1 out]
        n131 = Merge Errors(w343) -> (w346:errorcluster)
      }
      frame "Valid Optimizer" {
        # "When a Valid Optimizer has been chosen, start the other processes."
        n132 = Unbundle By Name(w353) -> ("Log Runs"=w352:bool)
        n133 = call "Enqueue Message (Single).vi"("error in (no error)"=w363, "Message Data"=w348, "Message"=w347, "Message Queue"=w350) -> ("error out"=w351:errorcluster, "dup Message Queue"=w349:refnum<queue>)  [unwired: 6 in]
        n134 = case shown="True" w352 {
          tunnel: w351 -> [w364 w368]
          tunnel: w349 -> [_ w367]
          tunnel: [w364 w365] -> w361
          frame False {
          }
          frame True {
            n135 = call "Enqueue Message (Single).vi"("error in (no error)"=w368, "Message"="Start", "Message Queue"=w367) -> ("error out"=w365:errorcluster)  [unwired: 7 in, 1 out]
          }
        }
        n136 = call "Enqueue Message (Single).vi"("error in (no error)"=w361, "Message"="Start", "Message Queue"=w360) -> ("error out"=w359:errorcluster)  [unwired: 7 in, 1 out]
        n137 = Unbundle By Name(w353) -> ("Clone"=w355:bool)
        n138 = call "Enqueue Message (Single).vi"("error in (no error)"=w359, "Message Data"=w348, "Message"=w347, "Message Queue"=w358) -> ("error out"=w356:errorcluster)  [unwired: 6 in, 1 out]
        n139 = case shown="False" w355 {
          tunnel: w356 -> [w372 w373]
          tunnel: [w371 w373] -> w354
          tunnel: w357 -> [w370 _]
          frame False {
            # "Show the Front Panel automatically on startup"
            n140 = call "Enqueue Message (Single).vi"("error in (no error)"=w372, "Message"="Show", "Message Queue"=w370) -> ("error out"=w371:errorcluster)  [unwired: 7 in, 1 out]
          }
          frame True {
            # "Reentrant clone. It is the responsibility of the RCM to send \"Show\"."
          }
        }
      }
      frame "Optimizer Started" {
        # "Notify processes of update"
        # "Build an array of all processes that will receive this message"
        # "Notify processes that the optimizer is running."
        n141 = Build Array(w375, w377, w376) -> (w374:refnum<queue>[])
        n142 = for {
          tunnel: w379 -> [w388]
          tunnel: w378 -> [w387]
          shift-right: [w385] -> w380
          shift-left: w382 -> [w384]
          tunnel: w374 -> [w386] mode=indexing
          n143 = call "Enqueue Message (Single).vi"("Message Data"=w388, "Message"=w387, "Message Queue"=w386) -> ("error out"=w383:errorcluster)  [unwired: 7 in, 1 out]
          n144 = Merge Errors(w383, w384) -> (w385:errorcluster)
        }
      }
      frame "Optimizer Stopped" {
        # "Exit program if the optimizer has failed"
        # "Build an array of all processes that will receive this message"
        # "Notify processes that the optimizer stopped."
        n145 = Build Array(w389) -> (w390:refnum<queue>[])
        n146 = for {
          shift-right: [w397] -> w391
          shift-left: w393 -> [w396]
          tunnel: w390 -> [w398] mode=indexing
          n147 = call "Enqueue Message (Single).vi"("Message"="Exit", "Message Queue"=w398) -> ("error out"=w395:errorcluster)  [unwired: 8 in, 1 out]
          n148 = Merge Errors(w395, w396) -> (w397:errorcluster)
        }
      }
      frame "Logging" {
        # "Enable or disable logging in the System Data. Run logging is disabled by default."
        n149 = Variant To Data(type=TRUE, Variant=w403) -> (data=w402:bool)  [unwired: 1 in, 1 out]
        n150 = case shown="True" w402 {
          tunnel: w401 -> [w412 w417]
          tunnel: [w411 w416] -> w400
          tunnel: w399 -> [w410 w415]
          frame False {
            n151 = call "Enqueue Message (Single).vi"("Priority Message? (F)"=TRUE, "error in (no error)"=w412, "Message"="Stop", "Message Queue"=w410) -> ("error out"=w411:errorcluster)  [unwired: 6 in, 1 out]
          }
          frame True {
            n152 = call "Enqueue Message (Single).vi"("Priority Message? (F)"=TRUE, "error in (no error)"=w417, "Message"="Start", "Message Queue"=w415) -> ("error out"=w416:errorcluster)  [unwired: 6 in, 1 out]
          }
        }
        n153 = Bundle By Name(cluster=w407, "Log Runs"=w402) -> (w405:T8)
        n154 = Merge Errors(w400) -> (w406:errorcluster)
      }
      frame "Config Logging" {
        # "Pass on Config Logging message to Logging Loop."
        n155 = call "Enqueue Message (Single).vi"("error in (no error)"=w422, "Message Data"=w419, "Message"=w418, "Message Queue"=w420) -> ("error out"=w421:errorcluster)  [unwired: 6 in, 1 out]
        n156 = Merge Errors(w421) -> (w423:errorcluster)
      }
      frame "Set Log Directory" {
        # "Pass on log setting message to Logging Loop."
        n157 = call "Enqueue Message (Single).vi"("error in (no error)"=w429, "Message Data"=w426, "Message"=w425, "Message Queue"=w427) -> ("error out"=w428:errorcluster)  [unwired: 6 in, 1 out]
        n158 = Merge Errors(w428) -> (w430:errorcluster)
      }
      frame "Set Log File Prefix" {
        # "Pass on log setting message to Logging Loop."
        n159 = call "Enqueue Message (Single).vi"("error in (no error)"=w436, "Message Data"=w433, "Message"=w432, "Message Queue"=w434) -> ("error out"=w435:errorcluster)  [unwired: 6 in, 1 out]
        n160 = Merge Errors(w435) -> (w437:errorcluster)
      }
      frame "Set Log File Delimiter" {
        # "Pass on log setting message to Logging Loop."
        n161 = call "Enqueue Message (Single).vi"("error in (no error)"=w443, "Message Data"=w440, "Message"=w439, "Message Queue"=w441) -> ("error out"=w442:errorcluster)  [unwired: 6 in, 1 out]
        n162 = Merge Errors(w442) -> (w444:errorcluster)
      }
      frame "Set Log on Run" {
        # "Pass on log setting message to Logging Loop."
        n163 = call "Enqueue Message (Single).vi"("error in (no error)"=w450, "Message Data"=w447, "Message"=w446, "Message Queue"=w448) -> ("error out"=w449:errorcluster)  [unwired: 6 in, 1 out]
        n164 = Merge Errors(w449) -> (w451:errorcluster)
      }
      frame "Logging Started" {
        # "Pass on Logging Started message to RCM and UI."
        n165 = Build Array(w454, w455) -> (w453:refnum<queue>[])
        n166 = for {
          tunnel: w457 -> [w464]
          tunnel: w456 -> [w463]
          shift-right: [w465] -> w458
          shift-left: w459 -> [w466]
          tunnel: w453 -> [w462] mode=indexing
          n167 = call "Enqueue Message (Single).vi"("error in (no error)"=w466, "Message Data"=w464, "Message"=w463, "Message Queue"=w462) -> ("error out"=w465:errorcluster)  [unwired: 6 in, 1 out]
        }
        n168 = Merge Errors(w458) -> (w460:errorcluster)
      }
      frame "Logging Stopped" {
        # "Pass on Logging Stopped message to RCM and UI."
        n169 = Build Array(w468, w469) -> (w467:refnum<queue>[])
        n170 = for {
          tunnel: w471 -> [w478]
          tunnel: w470 -> [w477]
          shift-right: [w479] -> w472
          shift-left: w473 -> [w480]
          tunnel: w467 -> [w476] mode=indexing
          n171 = call "Enqueue Message (Single).vi"("error in (no error)"=w480, "Message Data"=w478, "Message"=w477, "Message Queue"=w476) -> ("error out"=w479:errorcluster)  [unwired: 6 in, 1 out]
        }
        n172 = Merge Errors(w472) -> (w474:errorcluster)
      }
      frame "Submit Yield" {
        # "Forward the Submit Yield command to the OML and acquisition."
        n173 = Build Array(w482, w484, w481) -> (w483:refnum<queue>[])
        n174 = for {
          tunnel: w486 -> [w493]
          tunnel: w485 -> [w492]
          shift-right: [w494] -> w487
          shift-left: w490 -> [w495]
          tunnel: w483 -> [w491] mode=indexing
          n175 = call "Enqueue Message (Single).vi"("error in (no error)"=w495, "Message Data"=w492, "Message"=w493, "Message Queue"=w491) -> ("error out"=w494:errorcluster)  [unwired: 6 in, 1 out]
        }
        n176 = Merge Errors(w487) -> (w488:errorcluster)
      }
      frame "Flow Rate Changed" {
        # "Forward the Flow Rate Changed command to the OML and acquisition."
        n177 = Build Array(w497, w496) -> (w498:refnum<queue>[])
        n178 = for {
          tunnel: w500 -> [w507]
          tunnel: w499 -> [w506]
          shift-right: [w508] -> w501
          shift-left: w504 -> [w509]
          tunnel: w498 -> [w505] mode=indexing
          n179 = call "Enqueue Message (Single).vi"("error in (no error)"=w509, "Message Data"=w506, "Message"=w507, "Message Queue"=w505) -> ("error out"=w508:errorcluster)  [unwired: 6 in, 1 out]
        }
        n180 = Merge Errors(w501) -> (w502:errorcluster)
      }
      frame "Report" {
        # "Send instrument state notification"
        # "Notify processes of update"
        # "Notify processes that the instrument stopped running."
        n181 = Variant To Data(type=T2 {"Context"=refnum, "Socket"=refnum, "Running Since"=timestamp(0 s since 1904-01-01), "New Parameters (values)"={"Time Stamp"=timestamp(0 s since 1904-01-01), "Name"=[], "Value"=[]}, "Optimizer Path"=path "", "Running"=FALSE, "Response Counter"=0, "Response Timeout (ms)"=0, "Response Retries"=0, "Endpoint"="", "Starting up?"=FALSE, "New Parameters (percents)"={"Time Stamp"=timestamp(0 s since 1904-01-01), "Name"=[], "Value"=[]}, "Flow Rate Constant"=0.0, "Yield"=0.0, "Current Best (values)"={"Parameter Names"=[], "Parameter Values"=[], "Function Value"=0.0}} ("Instrument State"), Variant=w514) -> (data=w517:T2)  [unwired: 1 in, 1 out]
        n182 = Enqueue Element(queue=w518, element=w517) -> (error out=w515:errorcluster)  [unwired: 2 in, 2 out]
        n183 = Send Notification(notification=w517, notifier=w521) -> (error out=w519:errorcluster)  [unwired: 1 in, 1 out]
        n184 = Merge Errors(w515, w519) -> (w516:errorcluster)
        n185 = call "Enqueue Message (Single).vi"("Message Data"=w514, "Message"=w513, "Message Queue"=w512) -> ("error out"=w511:errorcluster)  [unwired: 7 in, 1 out]
        n186 = call "Enqueue Message (Single).vi"("Message Data"=w514, "Message"=w513, "Message Queue"=w523) -> ("error out"=w510:errorcluster)  [unwired: 7 in, 1 out]
        n187 = Merge Errors(w510, w511, w516) -> (w524:errorcluster)
      }
    }
    n188 = call "Error Handler - System Control Loop.vi"("error in (no error)"=w217, "Message Queue"=w219) -> ("dup error in"=w218:errorcluster)  [unwired: 8 in, 1 out]
  }
  n189 = call "Logging Message Loop.vi"("System Control"=w5, "Data Queue"=w7, "Logging"=w31) -> ("error out"=w16:errorcluster)  [unwired: 8 in]
  n190 = Unregister For Events(event registration refnum=w23) -> (error out=w18:errorcluster)  [unwired: 1 in]
  n191 = Merge Errors(w27, w19, w18, w17, w16, w15, w14) -> (w12:errorcluster)
  n192 = call <vilib>:"Simple Error Handler.vi"("error in (no error)"=w12) -> ()  [unwired: 4 in, 5 out]
  n193 = Cluster To Array(cluster=w11) -> (array=w10:refnum<queue>[])
  n194 = for {
    shift-right: [w526] -> w9
    shift-left: w12 -> [w527]
    tunnel: w10 -> [w528] mode=indexing
    n195 = Release Queue(queue=w528, force destroy? (F)=TRUE, error in (no error)=w527) -> (error out=w526:errorcluster)  [unwired: 2 out]
  }
  n196 = call "Destroy User Event - Stop.vi"("error in (no error)"=w9, "User Event - Stop"=w22) -> ("error out"=w24:errorcluster)  [unwired: 9 in]
  n197 = disable-structure shown="RUN_TIME_ENGINE==True" {
    disable-tunnel: w24 -> [_ _]
    frame condition #0 (active) {
    }
    frame condition #1 {
      # "Call Quit LabVIEW if running as a built application."
      n198 = Quit LabVIEW() -> ()  [unwired: 1 in]
    }
  }
